vi "Web Redirect Parameter Parser - Return.vi"(0 "redirect URL":string="Return_Success.httml", 1 "Device":T1, 3 "error in (no error)":errorcluster) -> (7 "Output String":string, 10 "error out":errorcluster)   [LabVIEW 2016]
uses:
  Device Info.ctl
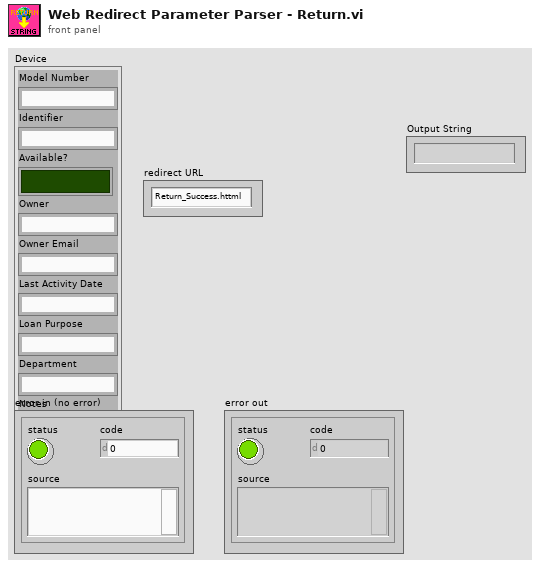
[diagram p1: front panel]
types:
  T1 = typedef "Device Info.ctl" = cluster{"Model Number":string, "Identifier":string, "Available?":bool, "Owner":string, "Owner Email":string, "Last Activity Date":string, "Loan Purpose":string, "Department":string, "Notes":string, "Serial Number":string}
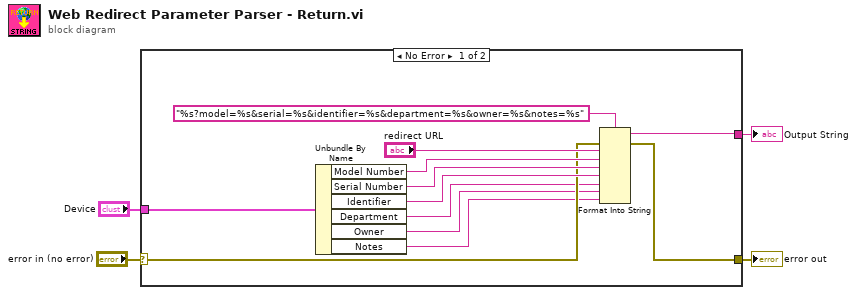
[diagram p0: block diagram]
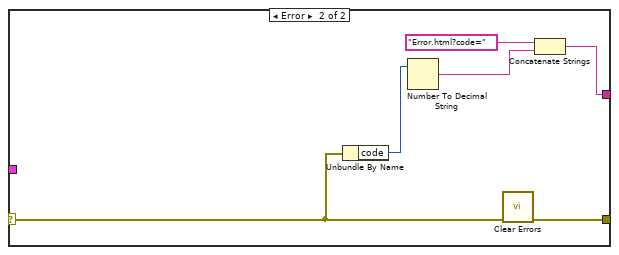
[diagram p2: hidden frame]
diagram:
  n1 = case shown="No Error" "error in (no error)" {
    selector: "error in (no error)" -> [w9 w21]
    tunnel: [w8 w22] -> w3
    tunnel: "Device" -> [w16 _]
    tunnel: [w10 w17] -> w1
    frame No Error {
      n2 = Unbundle By Name(w16) -> ("Model Number"=w13:string, "Serial Number"=w12:string, "Identifier"=w11:string, "Department"=w7:string, "Owner"=w6:string, "Notes"=w5:string)
      n3 = Format Into String(format string="%s?model=%s&serial=%s&identifier=%s&department=%s&owner=%s&notes=%s" ("initial string"), error in=w9, "redirect URL", w13, w12, w11, w7, w6, w5) -> (resulting string=w10:string, error out=w8:errorcluster)  [unwired: 1 in]
    }
    frame Error {
      n4 = Unbundle By Name(w21) -> ("code"=w20:i32)
      n5 = Number To Decimal String(number=w20) -> (decimal integer string=w18:string)  [unwired: 1 in]
      n6 = call <vilib>:"Clear Errors.vi"("error in (no error)"=w21) -> ("error out"=w22:errorcluster)  [unwired: 5 in, 1 out]
      n7 = Concatenate Strings("Error.html?code=", w18) -> (w17:string)
    }
  }
  "error out" <- w3
  "Output String" <- w1
